vi "angle.vi"(9 "Lidar Vertical Position":i8, 10 "Lidar Distance":u16, 11 "Lidar Scan Angle":u8) -> (0 "Robot Z":fxp<+/-,18,18>, 1 "Lidar Y":fxp<+/-,17,17>, 2 "Lidar X = Robot X":fxp<+/-,17,17>, 3 "Distance Object":fxp<+,38,18> format="%.26g", 4 "Is object?":bool, 5 "Robot Y":fxp<+/-,18,18>)   [LabVIEW 2009]
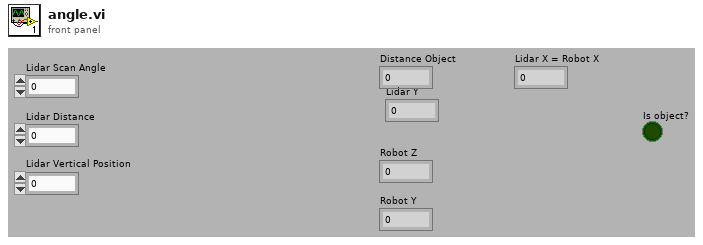
[diagram p1: front panel]
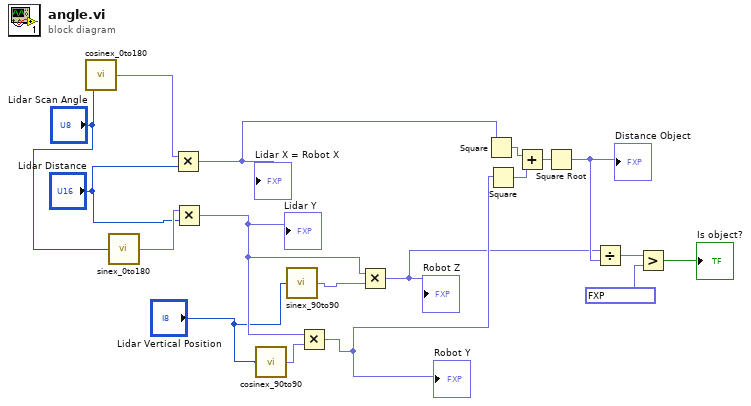
[diagram p0: block diagram]
diagram:
  n1 = call "cosinex_0to180.vi"("theta"="Lidar Scan Angle") -> ("Numeric"=w8:fxp<+/-,16,1>)
  n2 = call "sinex_0to180.vi"("theta"="Lidar Scan Angle") -> ("Numeric"=w7:fxp<+/-,16,1>)
  n3 = Multiply(x=w8, y="Lidar Distance") -> (x*y=w17:fxp<+/-,17,17>)
  "Lidar X = Robot X" <- w17
  n4 = Multiply(x=w7, y="Lidar Distance") -> (x*y=w18:fxp<+/-,17,17>)
  "Lidar Y" <- w18
  n5 = call "cosinex_90to90.vi"("theta"="Lidar Vertical Position") -> ("Numeric"=w4:fxp<+/-,16,1>)
  n6 = call "sinex_90to90.vi"("theta"="Lidar Vertical Position") -> ("Numeric"=w3:fxp<+/-,16,1>)
  n7 = Multiply(x=w18, y=w4) -> (x*y=w16:fxp<+/-,18,18>)
  "Robot Y" <- w16
  n8 = Multiply(x=w18, y=w3) -> (x*y=w1:fxp<+/-,18,18>)
  "Robot Z" <- w1
  n9 = Square(x=w17) -> (x^2=w13:fxp<+,33,33>)
  n10 = Square(x=w16) -> (x^2=w14:fxp<+,35,35>)
  n11 = Add(x=w13, y=w14) -> (x+y=w15:fxp<+,35,35>)
  n12 = Square Root(x=w15) -> (sqrt(x)=w12:fxp<+,38,18>)
  "Distance Object" <- w12
  n13 = Divide(x=w1, y=w12) -> (x/y=w11:fxp<+/-,56,38>)
  n14 = Greater?(x=w11, y=fxp<+,8,-2> 0.150390625) -> (0:→"Is object?":bool)
